vi "FTW-Endpoint-Tell.vi"(0 "FTW Endpoint":refnum<class "FTW-Endpoint-Notifier.lvclass">, 5 "Message Header":string, 7 "Message Body":string, 9 "Timeout":i32 format="%dmsec", 11 "error in":errorcluster) -> (4 "FTW Endpoint out":refnum<class "FTW-Endpoint-Notifier.lvclass">, 6 "Timed out?":bool, 15 "error out":errorcluster)   [LabVIEW 2013, in "FTW-Actor.lvlib" / "FTW-Endpoint-Notifier.lvclass"]
uses:
  FTW-Endpoint-Notifier.lvclass
panel:
  # "Inputs"
  # "Outputs"
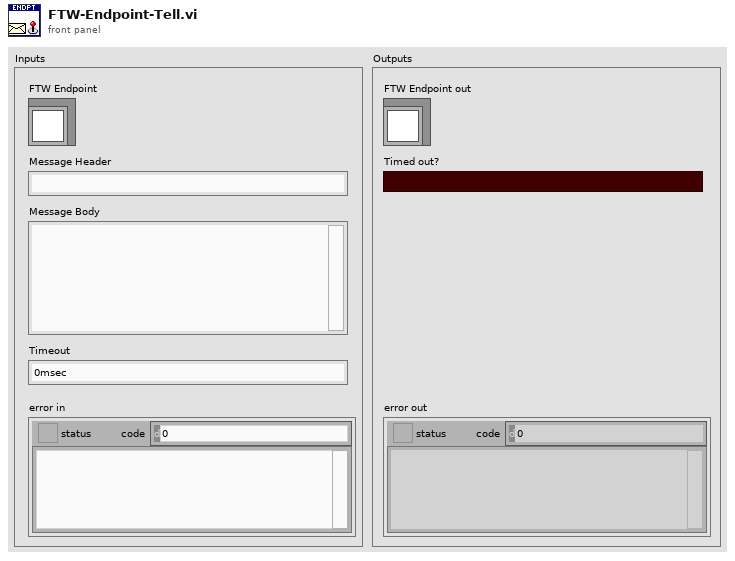
[diagram p1: front panel]
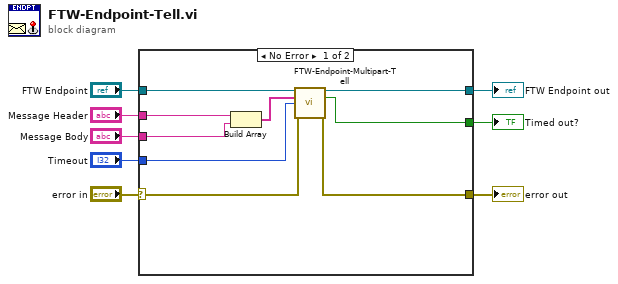
[diagram p0: block diagram]
diagram:
  n1 = case shown="No Error" "error in" {
    selector: "error in" -> [w15 w19]
    tunnel: [w14 w19] -> w8
    tunnel: [w16 w18] -> w6
    tunnel: "FTW Endpoint" -> [w17 w18]
    tunnel: [w9 _] -> w4
    tunnel: "Timeout" -> [w13 _]
    tunnel: "Message Header" -> [w12 _]
    tunnel: "Message Body" -> [w11 _]
    frame No Error {
      n2 = Build Array(w12, w11) -> (w10:string[])
      n3 = call-dynamic "FTW-Endpoint-Multipart-Tell.vi"("FTW Endpoint"=w17, "Multipart Message"=w10, "Timeout"=w13, "error in"=w15) -> ("FTW Endpoint out"=w16:refnum<class "FTW-Endpoint-Notifier.lvclass">, "Timed out?"=w9:bool, "error out"=w14:errorcluster)  [unwired: 9 in]
    }
    frame Error {
    }
  }
  "error out" <- w8
  "FTW Endpoint out" <- w6
  "Timed out?" <- w4
